vi "Configure Serial Baud Rate.vi"(8 "error in (no error)":errorcluster, 10 "Serial Configuration (19200 : 19200 Baud)":u32(ring)=19200 items=["19200"=19200, "57600"=57600, "115200"=115200, "250000"=250000, "500000"=500000, "750000"=750000], 11 "VISA resource name":refnum<visa-resource-name>) -> (0 "error out":errorcluster, 3 "VISA resource name out":refnum<visa-resource-name>)   [LabVIEW 2011, in "Hokuyo URG Series.lvlib"]
doc: "This VI changes the baud rate of the serial connection. When the device is connected using both serial and USB, the USB connection has priority and serial is not used. A command error might be returned if this command is called on an instrument that is not using a serial interface."
uses:
  Hokuyo URG Series.lvlib
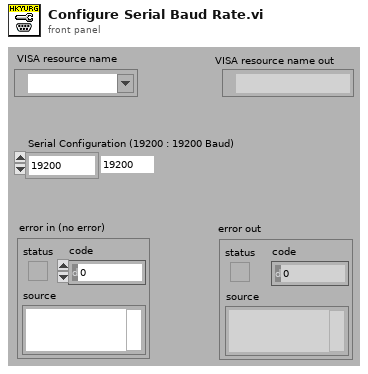
[diagram p1: front panel]
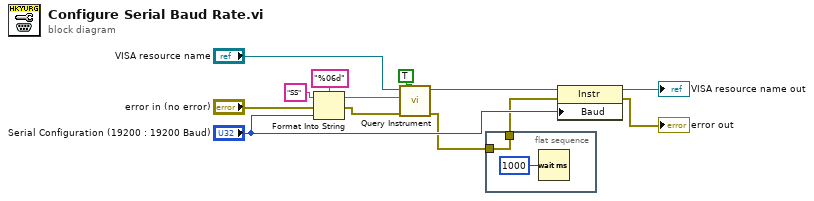
[diagram p0: block diagram]
diagram:
  n1 = Format Into String(format string="%06d", initial string="SS", error in="error in (no error)", "Serial Configuration (19200 : 19200 Baud)") -> (resulting string=w12:string, error out=w11:errorcluster)
  n2 = call "Query Instrument.vi"("Error Query (Enabled)"=TRUE, "error in"=w11, "Command"=w12, "VISA Resource Name"="VISA resource name") -> ("error out"=w2:errorcluster, "VISA Resource Name Out"=w5:refnum<visa-resource-name>)  [unwired: 5 in, 1 out]
  n3 = flat-sequence {
    tunnel: w2 -> [w14]
    tunnel: [w14] -> w1
    frame #0 {
      n4 = Wait (ms)(milliseconds to wait=u32 1000) -> ()  [unwired: 1 out]
    }
  }
  n5 = property class="Instr"(reference=w5, error in=w1, "Baud"="Serial Configuration (19200 : 19200 Baud)") -> (reference out=→"VISA resource name out":refnum<visa-resource-name>, error out=→"error out":errorcluster)
